vi "0_StaveSurvey.vi"(4 "Nloops":i32=1, 5 "Folder name for survey results":string, 6 "Axes Speeds [mm/s]":T2={"X Speed"=10.0, "Y Speed"=10.0, "Z Speed"=10.0}, 7 "Records directory":path=path "C:/Users/Aerotech/Documents/Stave Assembly Records/2017-03-30/ChangeHeight/corners.csv", 8 "error in (no error)":errorcluster, 9 "double( Time, Temp )":dbl[](array[numeric]), 10 "Most recently collected image":T4(plugin-control)=refnum, 11 "XYZ Stage .NET Refnum in":refnum<k24>) -> (0 "Error report":errorcluster, 3 "XYZ Stage .NET Refnum out":refnum<k24>)   [LabVIEW 2016]
uses:
  C:/Users/sciollalab/Documents/Brandeis-BNL/LabVIEW_Codes/BNLStaveAssembly-Blueprint/Bin/Aerotech.A3200.dll
  BNLStaveAssembly-Blueprint/Bin/Aerotech.A3200.dll
  <vilib>/Utility/file.llb/Read Delimited Spreadsheet (DBL).vi
  <vilib>/Utility/file.llb/Write Delimited Spreadsheet (DBL).vi
  <vilib>/regexp/Match Regular Expression.xnode
panel:
  in  "Tab Control":T1(tab)
  in  "File delimiter":string=","
  out "XYZ Stage Current Position":T3={"X [-750, 750 mm]"=122.51800503908298, "Y [-150, 150 mm]"=-145.62509155644523, "Z [-50, 50 mm]"=10.9688762056}
  in  "Wait before image capture [ms]":u32=5000
  out "Image #":i32=319
  out "Set of Coordinates to Process":dbl[][](array[numeric])=[[122.518, -50.0451, 9.5689], [122.518, -50.0451, 9.5689], [122.518, -50.0451, 9.5689], [122.518, -50.0451, 9.5689], [122.518, -50.0451, 9.5689], [122.518, -50.0451, 9.5689], [122.518, -50.0451, 9.5689], [122.518, -50.0451, 9.5689], [122.518, -50.0451, 9.5689], [122.518, -50.0451, 9.5689], [122.518, -50.0451, 9.768899999999999], [122.518, -50.0451, 9.768899999999999], [122.518, -50.0451, 9.768899999999999], [122.518, -50.0451, 9.768899999999999], [122.518, -50.0451, 9.768899999999999], [122.518, -50.0451, 9.768899999999999], [122.518, -50.0451, 9.768899999999999], [122.518, -50.0451, 9.768899999999999], [122.518, -50.0451, 9.768899999999999], [122.518, -50.0451, 9.768899999999999], [122.518, -50.0451, 9.9689], [122.518, -50.0451, 9.9689], [122.518, -50.0451, 9.9689], [122.518, -50.0451, 9.9689], [122.518, -50.0451, 9.9689], [122.518, -50.0451, 9.9689], [122.518, -50.0451, 9.9689], [122.518, -50.0451, 9.9689], [122.518, -50.0451, 9.9689], [122.518, -50.0451, 9.9689], [122.518, -50.0451, 10.168899999999999], [122.518, -50.0451, 10.168899999999999], [122.518, -50.0451, 10.168899999999999], [122.518, -50.0451, 10.168899999999999], [122.518, -50.0451, 10.168899999999999], [122.518, -50.0451, 10.168899999999999], [122.518, -50.0451, 10.168899999999999], [122.518, -50.0451, 10.168899999999999], [122.518, -50.0451, 10.168899999999999], [122.518, -50.0451, 10.168899999999999], [122.518, -50.0451, 10.3689], [122.518, -50.0451, 10.3689], [122.518, -50.0451, 10.3689], [122.518, -50.0451, 10.3689], [122.518, -50.0451, 10.3689], [122.518, -50.0451, 10.3689], [122.518, -50.0451, 10.3689], [122.518, -50.0451, 10.3689], [122.518, -50.0451, 10.3689], [122.518, -50.0451, 10.3689], [122.518, -50.0451, 10.5689], [122.518, -50.0451, 10.5689], [122.518, -50.0451, 10.5689], [122.518, -50.0451, 10.5689], [122.518, -50.0451, 10.5689], [122.518, -50.0451, 10.5689], [122.518, -50.0451, 10.5689], [122.518, -50.0451, 10.5689], [122.518, -50.0451, 10.5689], [122.518, -50.0451, 10.5689], [122.518, -50.0451, 10.768899999999999], [122.518, -50.0451, 10.768899999999999], [122.518, -50.0451, 10.768899999999999], [122.518, -50.0451, 10.768899999999999], [122.518, -50.0451, 10.768899999999999], [122.518, -50.0451, 10.768899999999999], [122.518, -50.0451, 10.768899999999999], [122.518, -50.0451, 10.768899999999999], [122.518, -50.0451, 10.768899999999999], [122.518, -50.0451, 10.768899999999999], [122.518, -50.0451, 10.9689], [122.518, -50.0451, 10.9689], [122.518, -50.0451, 10.9689], [122.518, -50.0451, 10.9689], [122.518, -50.0451, 10.9689], [122.518, -50.0451, 10.9689], [122.518, -50.0451, 10.9689], [122.518, -50.0451, 10.9689], [122.518, -50.0451, 10.9689], [122.518, -50.0451, 10.9689], [218.098, -50.0451, 9.5689], [218.098, -50.0451, 9.5689], [218.098, -50.0451, 9.5689], [218.098, -50.0451, 9.5689], [218.098, -50.0451, 9.5689], [218.098, -50.0451, 9.5689], [218.098, -50.0451, 9.5689], [218.098, -50.0451, 9.5689], [218.098, -50.0451, 9.5689], [218.098, -50.0451, 9.5689], [218.098, -50.0451, 9.768899999999999], [218.098, -50.0451, 9.768899999999999], [218.098, -50.0451, 9.768899999999999], [218.098, -50.0451, 9.768899999999999], [218.098, -50.0451, 9.768899999999999], [218.098, -50.0451, 9.768899999999999], [218.098, -50.0451, 9.768899999999999], [218.098, -50.0451, 9.768899999999999], [218.098, -50.0451, 9.768899999999999], [218.098, -50.0451, 9.768899999999999], [218.098, -50.0451, 9.9689], [218.098, -50.0451, 9.9689], [218.098, -50.0451, 9.9689], [218.098, -50.0451, 9.9689], [218.098, -50.0451, 9.9689], [218.098, -50.0451, 9.9689], [218.098, -50.0451, 9.9689], [218.098, -50.0451, 9.9689], [218.098, -50.0451, 9.9689], [218.098, -50.0451, 9.9689], [218.098, -50.0451, 10.168899999999999], [218.098, -50.0451, 10.168899999999999], [218.098, -50.0451, 10.168899999999999], [218.098, -50.0451, 10.168899999999999], [218.098, -50.0451, 10.168899999999999], [218.098, -50.0451, 10.168899999999999], [218.098, -50.0451, 10.168899999999999], [218.098, -50.0451, 10.168899999999999], [218.098, -50.0451, 10.168899999999999], [218.098, -50.0451, 10.168899999999999], [218.098, -50.0451, 10.3689], [218.098, -50.0451, 10.3689], [218.098, -50.0451, 10.3689], [218.098, -50.0451, 10.3689], [218.098, -50.0451, 10.3689], [218.098, -50.0451, 10.3689], [218.098, -50.0451, 10.3689], [218.098, -50.0451, 10.3689], [218.098, -50.0451, 10.3689], [218.098, -50.0451, 10.3689], [218.098, -50.0451, 10.5689], [218.098, -50.0451, 10.5689], [218.098, -50.0451, 10.5689], [218.098, -50.0451, 10.5689], [218.098, -50.0451, 10.5689], [218.098, -50.0451, 10.5689], [218.098, -50.0451, 10.5689], [218.098, -50.0451, 10.5689], [218.098, -50.0451, 10.5689], [218.098, -50.0451, 10.5689], [218.098, -50.0451, 10.768899999999999], [218.098, -50.0451, 10.768899999999999], [218.098, -50.0451, 10.768899999999999], [218.098, -50.0451, 10.768899999999999], [218.098, -50.0451, 10.768899999999999], [218.098, -50.0451, 10.768899999999999], [218.098, -50.0451, 10.768899999999999], [218.098, -50.0451, 10.768899999999999], [218.098, -50.0451, 10.768899999999999], [218.098, -50.0451, 10.768899999999999], [218.098, -50.0451, 10.9689], [218.098, -50.0451, 10.9689], [218.098, -50.0451, 10.9689], [218.098, -50.0451, 10.9689], [218.098, -50.0451, 10.9689], [218.098, -50.0451, 10.9689], [218.098, -50.0451, 10.9689], [218.098, -50.0451, 10.9689], [218.098, -50.0451, 10.9689], [218.098, -50.0451, 10.9689], [218.098, -145.6251, 9.5689], [218.098, -145.6251, 9.5689], [218.098, -145.6251, 9.5689], [218.098, -145.6251, 9.5689], [218.098, -145.6251, 9.5689], [218.098, -145.6251, 9.5689], [218.098, -145.6251, 9.5689], [218.098, -145.6251, 9.5689], [218.098, -145.6251, 9.5689], [218.098, -145.6251, 9.5689], [218.098, -145.6251, 9.768899999999999], [218.098, -145.6251, 9.768899999999999], [218.098, -145.6251, 9.768899999999999], [218.098, -145.6251, 9.768899999999999], [218.098, -145.6251, 9.768899999999999], [218.098, -145.6251, 9.768899999999999], [218.098, -145.6251, 9.768899999999999], [218.098, -145.6251, 9.768899999999999], [218.098, -145.6251, 9.768899999999999], [218.098, -145.6251, 9.768899999999999], [218.098, -145.6251, 9.9689], [218.098, -145.6251, 9.9689], [218.098, -145.6251, 9.9689], [218.098, -145.6251, 9.9689], [218.098, -145.6251, 9.9689], [218.098, -145.6251, 9.9689], [218.098, -145.6251, 9.9689], [218.098, -145.6251, 9.9689], [218.098, -145.6251, 9.9689], [218.098, -145.6251, 9.9689], [218.098, -145.6251, 10.168899999999999], [218.098, -145.6251, 10.168899999999999], [218.098, -145.6251, 10.168899999999999], [218.098, -145.6251, 10.168899999999999], [218.098, -145.6251, 10.168899999999999], [218.098, -145.6251, 10.168899999999999], [218.098, -145.6251, 10.168899999999999], [218.098, -145.6251, 10.168899999999999], [218.098, -145.6251, 10.168899999999999], [218.098, -145.6251, 10.168899999999999], [218.098, -145.6251, 10.3689], [218.098, -145.6251, 10.3689], [218.098, -145.6251, 10.3689], [218.098, -145.6251, 10.3689], [218.098, -145.6251, 10.3689], [218.098, -145.6251, 10.3689], [218.098, -145.6251, 10.3689], [218.098, -145.6251, 10.3689], [218.098, -145.6251, 10.3689], [218.098, -145.6251, 10.3689], [218.098, -145.6251, 10.5689], [218.098, -145.6251, 10.5689], [218.098, -145.6251, 10.5689], [218.098, -145.6251, 10.5689], [218.098, -145.6251, 10.5689], [218.098, -145.6251, 10.5689], [218.098, -145.6251, 10.5689], [218.098, -145.6251, 10.5689], [218.098, -145.6251, 10.5689], [218.098, -145.6251, 10.5689], [218.098, -145.6251, 10.768899999999999], [218.098, -145.6251, 10.768899999999999], [218.098, -145.6251, 10.768899999999999], [218.098, -145.6251, 10.768899999999999], [218.098, -145.6251, 10.768899999999999], [218.098, -145.6251, 10.768899999999999], [218.098, -145.6251, 10.768899999999999], [218.098, -145.6251, 10.768899999999999], [218.098, -145.6251, 10.768899999999999], [218.098, -145.6251, 10.768899999999999], [218.098, -145.6251, 10.9689], [218.098, -145.6251, 10.9689], [218.098, -145.6251, 10.9689], [218.098, -145.6251, 10.9689], [218.098, -145.6251, 10.9689], [218.098, -145.6251, 10.9689], [218.098, -145.6251, 10.9689], [218.098, -145.6251, 10.9689], [218.098, -145.6251, 10.9689], [218.098, -145.6251, 10.9689], [122.518, -145.6251, 9.5689], [122.518, -145.6251, 9.5689], [122.518, -145.6251, 9.5689], [122.518, -145.6251, 9.5689], [122.518, -145.6251, 9.5689], [122.518, -145.6251, 9.5689], [122.518, -145.6251, 9.5689], [122.518, -145.6251, 9.5689], [122.518, -145.6251, 9.5689], [122.518, -145.6251, 9.5689], [122.518, -145.6251, 9.768899999999999], [122.518, -145.6251, 9.768899999999999], [122.518, -145.6251, 9.768899999999999], [122.518, -145.6251, 9.768899999999999], [122.518, -145.6251, 9.768899999999999], [122.518, -145.6251, 9.768899999999999], [122.518, -145.6251, 9.768899999999999], [122.518, -145.6251, 9.768899999999999], [122.518, -145.6251, 9.768899999999999], [122.518, -145.6251, 9.768899999999999], [122.518, -145.6251, 9.9689], [122.518, -145.6251, 9.9689], [122.518, -145.6251, 9.9689], [122.518, -145.6251, 9.9689], [122.518, -145.6251, 9.9689], [122.518, -145.6251, 9.9689], [122.518, -145.6251, 9.9689], [122.518, -145.6251, 9.9689], [122.518, -145.6251, 9.9689], [122.518, -145.6251, 9.9689], [122.518, -145.6251, 10.168899999999999], [122.518, -145.6251, 10.168899999999999], [122.518, -145.6251, 10.168899999999999], [122.518, -145.6251, 10.168899999999999], [122.518, -145.6251, 10.168899999999999], [122.518, -145.6251, 10.168899999999999], [122.518, -145.6251, 10.168899999999999], [122.518, -145.6251, 10.168899999999999], [122.518, -145.6251, 10.168899999999999], [122.518, -145.6251, 10.168899999999999], [122.518, -145.6251, 10.3689], [122.518, -145.6251, 10.3689], [122.518, -145.6251, 10.3689], [122.518, -145.6251, 10.3689], [122.518, -145.6251, 10.3689], [122.518, -145.6251, 10.3689], [122.518, -145.6251, 10.3689], [122.518, -145.6251, 10.3689], [122.518, -145.6251, 10.3689], [122.518, -145.6251, 10.3689], [122.518, -145.6251, 10.5689], [122.518, -145.6251, 10.5689], [122.518, -145.6251, 10.5689], [122.518, -145.6251, 10.5689], [122.518, -145.6251, 10.5689], [122.518, -145.6251, 10.5689], [122.518, -145.6251, 10.5689], [122.518, -145.6251, 10.5689], [122.518, -145.6251, 10.5689], [122.518, -145.6251, 10.5689], [122.518, -145.6251, 10.768899999999999], [122.518, -145.6251, 10.768899999999999], [122.518, -145.6251, 10.768899999999999], [122.518, -145.6251, 10.768899999999999], [122.518, -145.6251, 10.768899999999999], [122.518, -145.6251, 10.768899999999999], [122.518, -145.6251, 10.768899999999999], [122.518, -145.6251, 10.768899999999999], [122.518, -145.6251, 10.768899999999999], [122.518, -145.6251, 10.768899999999999], [122.518, -145.6251, 10.9689], [122.518, -145.6251, 10.9689], [122.518, -145.6251, 10.9689], [122.518, -145.6251, 10.9689], [122.518, -145.6251, 10.9689], [122.518, -145.6251, 10.9689], [122.518, -145.6251, 10.9689], [122.518, -145.6251, 10.9689], [122.518, -145.6251, 10.9689], [122.518, -145.6251, 10.9689]]
  # "STAVE SURVEY Brandeis University - Brookhaven National Laboratory * ATLAS Phase II Inner Tracker Upgrade"
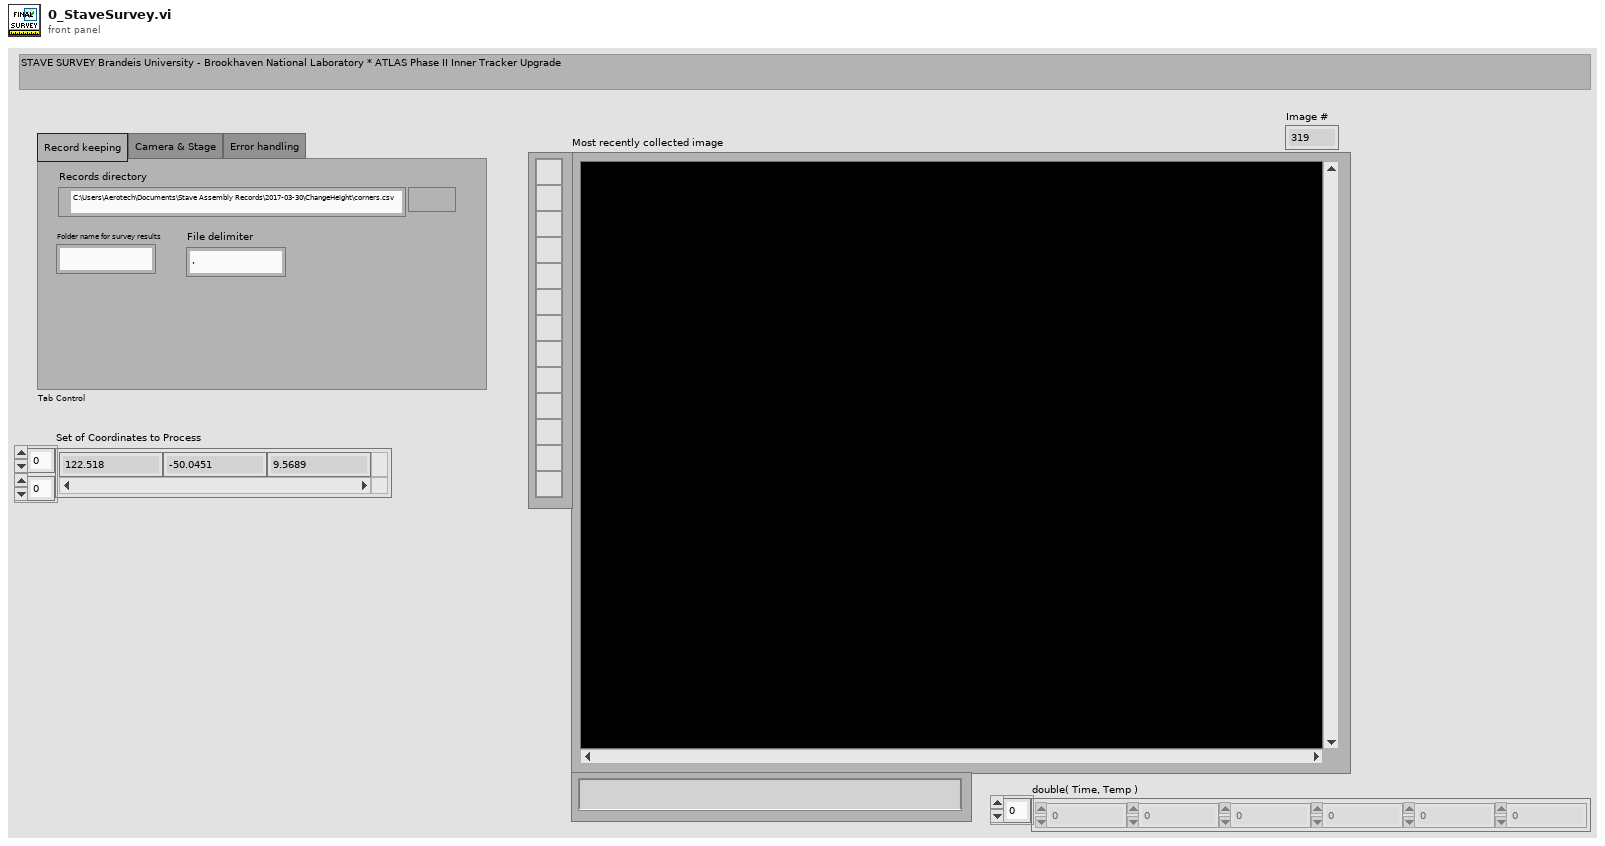
[diagram p1: front panel]
types:
  T1 = enum32{"Record keeping", "Camera & Stage", "Error handling"}
  T2 = cluster{"X Speed":dbl, "Y Speed":dbl, "Z Speed":dbl}
  T3 = cluster{"X [-750, 750 mm]":dbl, "Y [-150, 150 mm]":dbl, "Z [-50, 50 mm]":dbl}
  T4 = typedef "IMAQ Image.ctl" = refnum<image>
  T5 = cluster{"all rows[0]":dbl, "all rows[1]":dbl, "all rows[2]":dbl}
  T6 = cluster{"Final X":dbl, "Final Y":dbl, "Final Z":dbl}
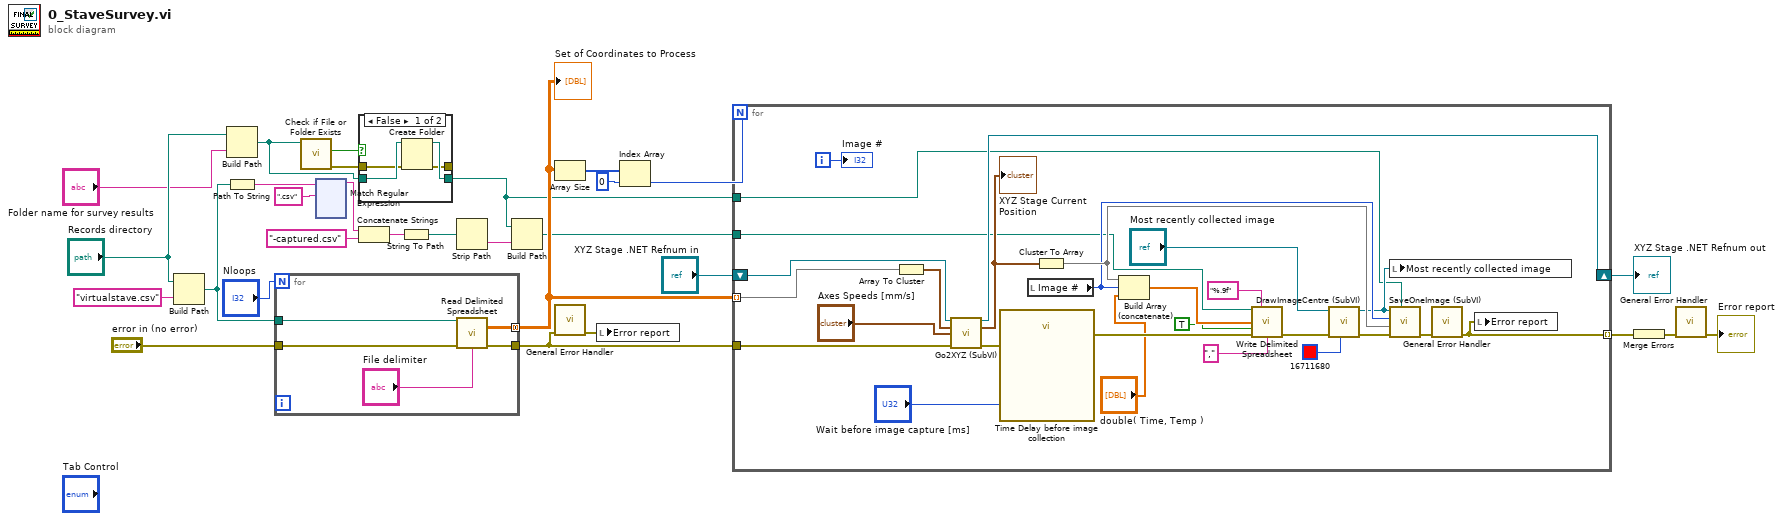
[diagram p0: block diagram]
diagram:
  n1 = Build Path(base path="Records directory", name or relative path="virtualstave.csv") -> (appended path=w1:path)
  n2 = Build Path(base path="Records directory", name or relative path="Folder name for survey results") -> (appended path=w13:path)
  n3 = Path To String(path=w1) -> (string=w6:string)
  n4 = for {
    N: "Nloops" -> [_]
    tunnel: w1 -> [w30]
    tunnel: [w31] -> w12 mode=concatenating
    tunnel: "error in (no error)" -> [w34]
    tunnel: [w32] -> w21
    n5 = call-poly <vilib>:"Read Delimited Spreadsheet.vi"("file path (dialog if empty)"=w30, "error in (no error)"=w34, "delimiter (\\t)"="File delimiter") -> ("all rows"=w31:dbl[][], "error out"=w32:errorcluster)  [unwired: 7 in, 4 out]
  }
  "Set of Coordinates to Process" <- w12
  n6 = call <vilib>:"Check if File or Folder Exists.vi"("path"=w13) -> ("error out"=w17:errorcluster, "file or folder exists?"=w16:bool)  [unwired: 8 in, 1 out]
  n7 = xnode "Match Regular Expression"("input string"=w6, "regular expression"=".csv") -> ("before match"=w9:string)  [unwired: 4 in, 4 out]
  n8 = case shown="False" w16 {
    tunnel: w13 -> [w38 w40]
    tunnel: [w37 w40] -> w2
    tunnel: w17 -> [w36 w39]
    tunnel: [w35 w39] -> _
    frame False {
      n9 = Create Folder(path (use dialog)=w38, error in=w36) -> (created path=w37:path, error out=w35:errorcluster)  [unwired: 1 in, 1 out]
    }
    frame True {
    }
  }
  n10 = Concatenate Strings(w9, "-captured.csv" ("name or relative path")) -> (w10:string)
  n11 = String To Path(string=w10) -> (path=w5:path)
  n12 = Strip Path(path=w5) -> (name=w4:string)  [unwired: 1 out]
  n13 = Build Path(base path=w2, name or relative path=w4) -> (appended path=w3:path)
  n14 = Array Size(array=w12) -> (size(s)=w22:i32[])
  n15 = call <vilib>:"General Error Handler.vi"("error in (no error)"=w21) -> ("error out"=w26:errorcluster)  [unwired: 2 in, 12 out]
  n16 = local write "Error report"(w26) -> ()
  n17 = Index Array(array=w22, index=0) -> (element=w28:i32)
  n18 = for {
    N: w28 -> [_]
    tunnel: w21 -> [w51]
    tunnel: [w44] -> w27 mode=indexing
    tunnel: w12 -> [w53] mode=indexing
    tunnel: w3 -> [w42]
    shift-right: [w49] -> w11
    shift-left: "XYZ Stage .NET Refnum in" -> [w66]
    tunnel: w2 -> [w43]
    i -> [w67]
    n19 = Array To Cluster(array=w53) -> (cluster=w52:T5)
    n20 = call "Go2XYZ (SubVI).vi"(".NET Refnum in"=w66, "Go to Coordinates"=w52, "Axis Speeds"="Axes Speeds [mm/s]", "error in (no error)"=w51) -> (".NET Refnum out"=w49:refnum<k24>, "Final Position"=w57:T6, "error out"=w50:errorcluster)  [unwired: 7 in, 2 out]
    "XYZ Stage Current Position" <- w57
    n21 = call "Time Delay before image collection"("error in (no error)"=w50, "Delay Time (s)"="Wait before image capture [ms]") -> ("error out"=w48:errorcluster)  [unwired: 9 in]
    n22 = local read "Image #"() -> (w64:i32)
    n23 = Cluster To Array(cluster=w57) -> (array=w65:dbl[])
    n24 = Build Array (concatenate)(w65, w64, "double( Time, Temp )") -> (w62:dbl[])
    n25 = call-poly <vilib>:"Write Delimited Spreadsheet.vi"("file path (dialog if empty)"=w42, "format (%.3f)"="%.9f", "1D data"=w62, "append to file? (new file:F)"=TRUE, "error in (no error)"=w48, "delimiter (\\t)"="," ("delimiter (\\t)")) -> ("error out"=w47:errorcluster)  [unwired: 8 in, 1 out]
    n26 = call "DrawImageCentre (SubVI).vi"("Axis colour"=u32 16711680, "error in (no error)"=w47, "Refnum in"="Most recently collected image") -> ("error out"=w46:errorcluster, "Refnum out"=w55:T4)  [unwired: 7 in]
    n27 = local write "Most recently collected image"(w55) -> ()
    n28 = call "SaveOneImage (SubVI).vi"("Save images path"=w43, "error in (no error)"=w46, "XYZ stage coordinates of image"=w65, "Image Number"=w64, "Image"=w55) -> ("error out"=w45:errorcluster)  [unwired: 6 in]
    n29 = call <vilib>:"General Error Handler.vi"("error in (no error)"=w45) -> ("error out"=w44:errorcluster)  [unwired: 2 in, 12 out]
    n30 = local write "Error report"(w44) -> ()
    "Image #" <- w67
  }
  "XYZ Stage .NET Refnum out" <- w11
  n31 = Merge Errors(w27) -> (w23:errorcluster)
  n32 = call <vilib>:"General Error Handler.vi"("error in (no error)"=w23) -> ("error out"=→"Error report":errorcluster)  [unwired: 2 in, 12 out]
